vi "Configure HF Reject Enabled.vi"(8 "error in (no error)":errorcluster {"code" format="%.0x"}, 10 "hf reject enabled (False)":bool caption="HF Reject Enabled (False)", 11 "VISA Resource Name":refnum<visa-resource-name>) -> (0 "error out":errorcluster {"code" format="%.0x"}, 3 "VISA Resource Name Out":refnum<visa-resource-name>)   [LabVIEW 2011, in "Agilent 546XX Series.lvlib"]
doc: "This VI specifies whether to apply trigger high frequency reject in its trigger circuit.\n\nNote: This VI is invalid when the trigger coupling specified by the VI ag546xx Configure Trigger Coupling is TV or LF Reject."
uses:
  Agilent 546XX Series.lvlib
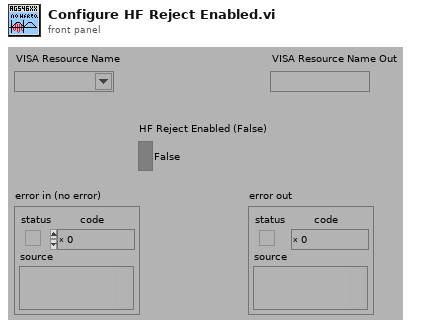
[diagram p1: front panel]
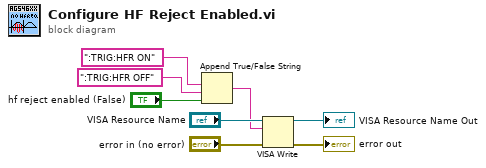
[diagram p0: block diagram]
diagram:
  n1 = Append True/False String(1:"hf reject enabled (False)", 2:":TRIG:HFR OFF" ("true string"), 3:":TRIG:HFR ON" ("true string")) -> (0:w4:string)  [unwired: 1 in]
  n2 = VISA Write(VISA resource name="VISA Resource Name", write buffer=w4, error in (no error)="error in (no error)") -> (VISA resource name out=→"VISA Resource Name Out":refnum<visa-resource-name>, error out=→"error out":errorcluster)  [unwired: 1 out]
